vi "TCP-CommError.vi"(0 "connection ID":refnum<k5>, 11 "error IN":errorcluster) -> (4 "CID Out":refnum<k5>, 8 "Boolean":bool, 15 "error OUT":errorcluster)   [LabVIEW 2011]
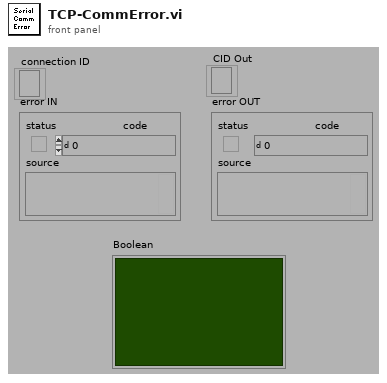
[diagram p1: front panel]
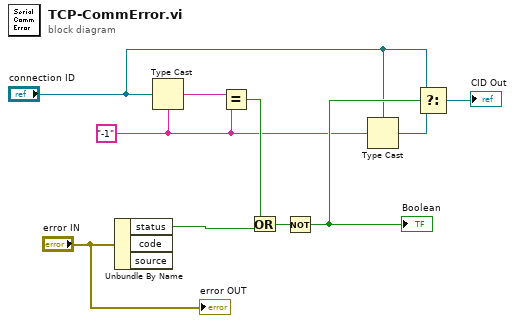
[diagram p0: block diagram]
diagram:
  w2 = "-1"
  n1 = Unbundle By Name("error IN") -> ("status"=w7:bool)  [unwired: 2 out]
  n2 = Type Cast(type=w2, x="connection ID") -> (*(type *) &x=w9:string)
  n3 = Equal?(x=w9, y=w2) -> (x = y?=w8:bool)
  n4 = Or(x=w8, y=w7) -> (x .or. y?=w6:bool)
  n5 = Not(x=w6) -> (.not. x?=w5:bool)
  "Boolean" <- w5
  n6 = Type Cast(type="connection ID", x=w2) -> (*(type *) &x=w3:refnum<k5>)
  n7 = Select(t="connection ID", s=w5, f=w3) -> (s? t:f=→"CID Out":refnum<k5>)
  "error OUT" <- "error IN"
